vi "Destroy User Define Events.vi"(8 "Error In":errorcluster, 11 "BNT_XtGraph in":refnum<class "BNT_XtGraph.lvclass">) -> (0 "Error Out":errorcluster, 3 "BNT_XtGraph out":refnum<class "BNT_XtGraph.lvclass">)   [LabVIEW 2019, in "BNT_XtGraph.lvlib" / "BNT_XtGraph.lvclass"]
doc: "Destroy all user defined events."
uses:
  BNT_XtGraph.lvclass
  BNT_XtGraph.lvclass/BNT_XtGraph.ctl
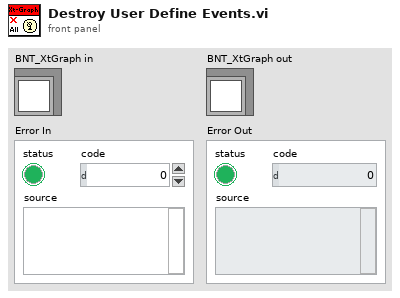
[diagram p1: front panel]
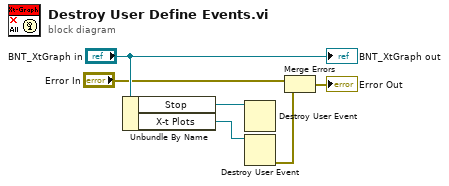
[diagram p0: block diagram]
diagram:
  n1 = Unbundle By Name("BNT_XtGraph in") -> ("Stop"=w1:refnum<user-event>, "X-t Plots"=w6:refnum<user-event>)
  n2 = Destroy User Event(user event=w1) -> ()  [unwired: 1 in, 1 out]
  n3 = Destroy User Event(user event=w6) -> (error out=w4:errorcluster)  [unwired: 1 in]
  n4 = Merge Errors("Error In", w4) -> (→"Error Out":errorcluster)
  "BNT_XtGraph out" <- "BNT_XtGraph in"
